vi "Read Fixture ID.vi"(8 "error in (no error)":errorcluster, 11 "LunchTest in":refnum<class "LunchTest.lvclass">) -> (0 "error out":errorcluster, 2 "Fixture ID":string[](array[string]), 3 "LunchTest out":refnum<class "LunchTest.lvclass">)   [LabVIEW 2019, in "SignalProcessing.lvlib" / "LunchTest.lvclass"]
uses:
  LunchTest.lvclass
  LunchTest.lvclass/LunchTest.ctl
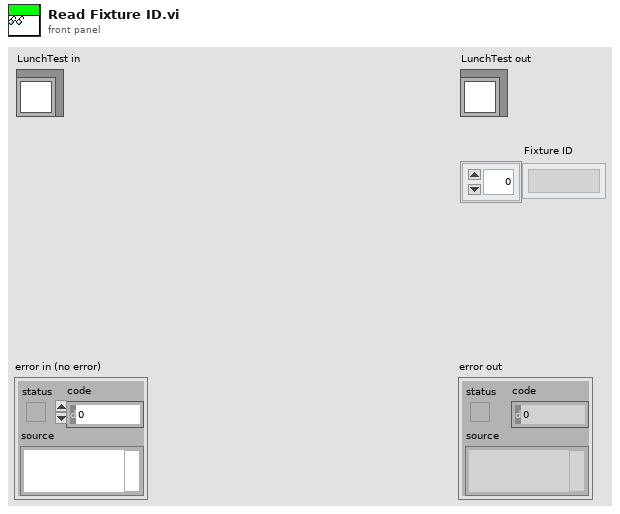
[diagram p1: front panel]
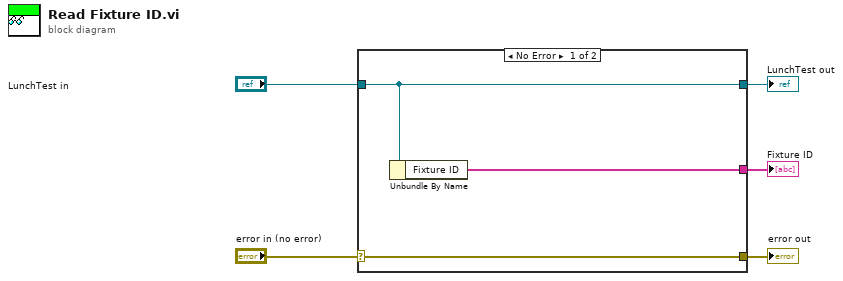
[diagram p0: block diagram]
diagram:
  n1 = case shown="No Error" "error in (no error)" {
    selector: "error in (no error)" -> [w8 w9]
    tunnel: [w8 w9] -> w4
    tunnel: [w7 w10] -> w2
    tunnel: "LunchTest in" -> [w7 w10]
    tunnel: [w6 _] -> w1
    frame No Error {
      n2 = Unbundle By Name(w7) -> ("Fixture ID"=w6:string[])
    }
    frame Error {
    }
  }
  "error out" <- w4
  "LunchTest out" <- w2
  "Fixture ID" <- w1
